vi "Get Bucket Notification Configuration.vi"(4 "Region":T1, 8 "error in (no error)":errorcluster, 9 "Bucket":string) -> (0 "error out":errorcluster, 3 "NotificationConfiguration":T2)   [LabVIEW 2015, in "LV Interface for Amazon S3.lvlib"]
doc: "This operation <B>returns the notification configuration</B> of a bucket. If notifications are not enabled on the bucket, the operation returns an empty NotificatonConfiguration element. <B>You must be the bucket owner to read the notification configuration</B> of a bucket. The bucket owner can use a bucket policy to grant permission to other users to read this configuration with the s3:GetBucketNotification permission."
uses:
  LV Interface for Amazon S3.lvlib
  Typedefs/AMZ_S3_NotificationConfiguration.ctl
  Typedefs/AMZ_S3_CompleteTopicConfiguration.ctl
  Typedefs/AMZ_S3_Event.ctl
  Typedefs/AMZ_S3_FilterRule.ctl
  Typedefs/AMZ_S3_CloudFunctionConfiguration.ctl
  Typedefs/AMZ_S3_QueueConfiguration.ctl
  Typedefs/AMZ_S3_LocationConstraint.ctl
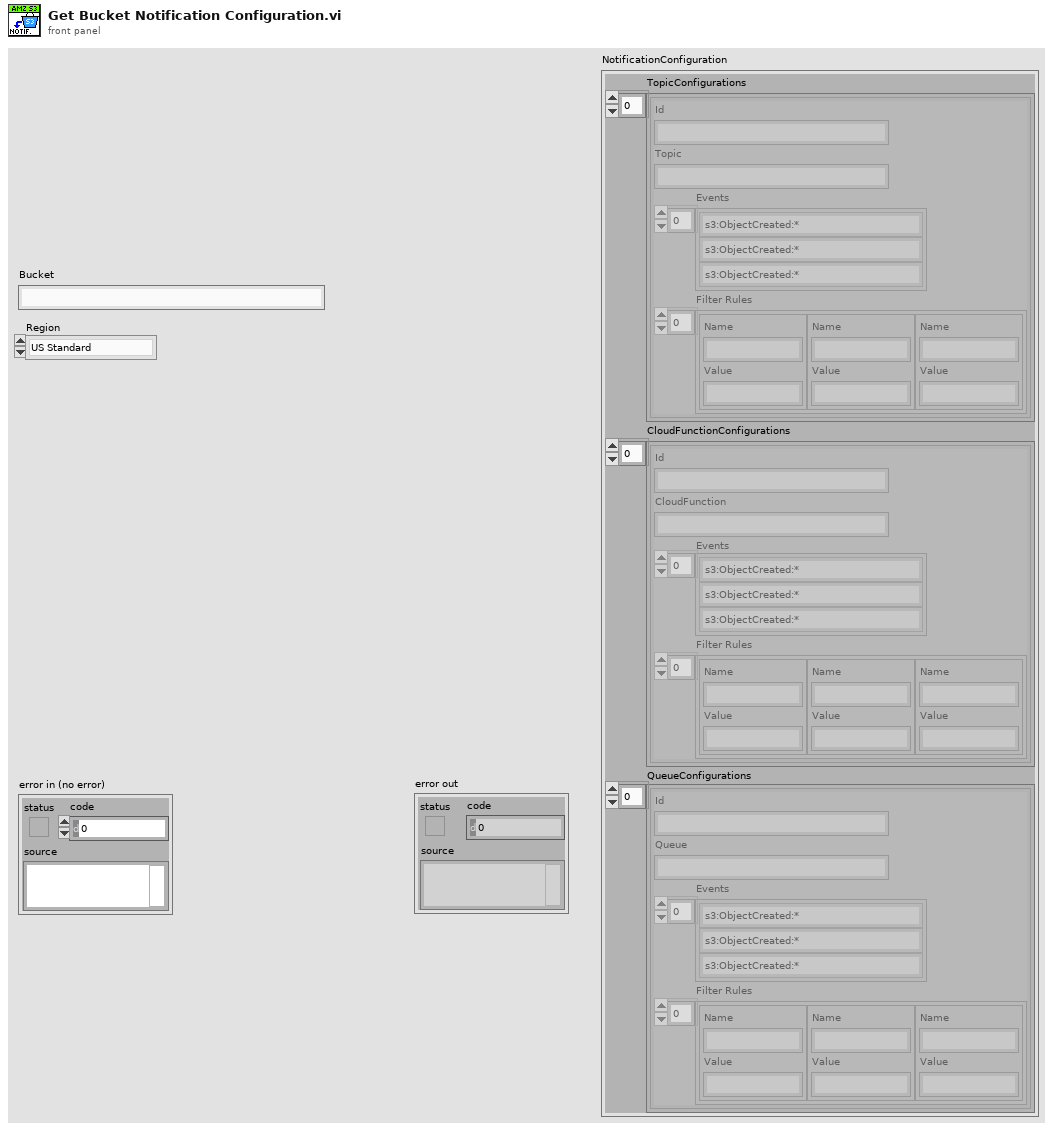
[diagram p1: front panel]
types:
  T1 = typedef "LV Interface for Amazon S3.lvlib/AMZ_S3_LocationConstraint.ctl" = enum16{"US Standard", "us-east-2", "us-west-1", "us-west-2", "ap-northeast-1", "ap-northeast-2", "ap-southeast-1", "ap-southeast-2", "ca-central-1", "eu-central-1", "eu-west-1", "eu-west-2", "sa-east-1"}
  T2 = typedef "LV Interface for Amazon S3.lvlib/AMZ_S3_NotificationConfiguration.ctl" = cluster{"TopicConfigurations":T3[], "CloudFunctionConfigurations":T6[], "QueueConfigurations":T7[]}
  T3 = typedef "LV Interface for Amazon S3.lvlib/AMZ_S3_CompleteTopicConfiguration.ctl" = cluster{"Id":string, "Topic":string, "Events":T4[], "Filter Rules":T5[]}
  T4 = typedef "LV Interface for Amazon S3.lvlib/AMZ_S3_Event.ctl" = enum16{"s3:ObjectCreated:*", "s3:ObjectCreated:Put", "s3:ObjectCreated:Post", "s3:ObjectCreated:Copy", "s3:ObjectCreated:CompleteMultipartUpload", "s3:ObjectRemoved:*", "s3:ObjectRemoved:Delete", "s3:ObjectRemoved:DeleteMarkerCreated", "s3:ReducedRedundancyLostObject"}
  T5 = typedef "LV Interface for Amazon S3.lvlib/AMZ_S3_FilterRule.ctl" = cluster{"Name":string, "Value":string}
  T6 = typedef "LV Interface for Amazon S3.lvlib/AMZ_S3_CloudFunctionConfiguration.ctl" = cluster{"Id":string, "CloudFunction":string, "Events":T4[], "Filter Rules":T5[]}
  T7 = typedef "LV Interface for Amazon S3.lvlib/AMZ_S3_QueueConfiguration.ctl" = cluster{"Id":string, "Queue":string, "Events":T4[], "Filter Rules":T5[]}
  T8 = typedef "LV Interface for Amazon S3.lvlib/AMZ_S3_Call Results.ctl" = enum16{"Success", "UndefinedError", "AccessDenied", "AccountProblem", "AmbiguousGrantByEmailAddress", "BadDigest", "BucketAlreadyExists", "BucketAlreadyOwnedByYou", "BucketNotEmpty", "CredentialsNotSupported", "CrossLocationLoggingProhibited", "EntityTooSmall", "EntityTooLarge", "ExpiredToken", "IllegalVersioningConfigurationException", "IncompleteBody", "IncorrectNumberOfFilesInPostRequest", "InlineDataTooLarge", "InternalError", "InvalidAccessKeyId", "InvalidAddressingHeader", "InvalidArgument", "InvalidBucketName", "InvalidDigest", "InvalidLocationConstraint", "InvalidPart", "InvalidPartOrder", "InvalidPayer", "InvalidPolicyDocument", "InvalidRange", "InvalidSecurity", "InvalidSOAPRequest", "InvalidStorageClass", "InvalidTargetBucketForLogging", "InvalidToken", "InvalidURI", "KeyTooLong", "MalformedACLError", "MalformedPOSTRequest", "MalformedXML", "MaxMessageLengthExceeded", "MaxPostPreDataLengthExceededError", "MetadataTooLarge", "MethodNotAllowed", "MissingAttachment", "MissingContentLength", "MissingRequestBodyError", "MissingSecurityElement", "MissingSecurityHeader", "NoLoggingStatusForKey", "NoSuchBucket", "NoSuchKey", "NoSuchUpload", "NoSuchVersion", "NotImplemented", "NotSignedUp", "OperationAborted", "PermanentRedirect", "PreconditionFailed", "Redirect", "RequestIsNotMultiPartContent", "RequestTimeout", "RequestTimeTooSkewed", "RequestTorrentOfBucketError", "SignatureDoesNotMatch", "SlowDown", "TemporaryRedirect", "TokenRefreshRequired", "TooManyBuckets", "UnexpectedContent", "UnresolvableGrantByEmailAddress", "UserKeyMustBeSpecified", "LabVIEWError"}
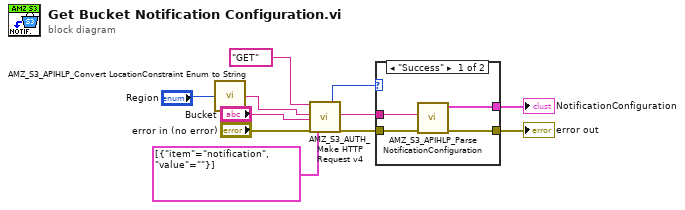
[diagram p0: block diagram]
diagram:
  n1 = call "AMZ_S3_APIHLP_Convert LocationConstraint Enum to String.vi"("Location"="Region") -> ("Location String"=w1:string)  [unwired: 4 in]
  n2 = call "AMZ_S3_AUTH_Make HTTP Request v4.vi"("HTTP-Verb"="GET", "Region"=w1, "Bucket"="Bucket", "error in"="error in (no error)", "request parameters"=cluster{"item":string, "value":string}[] [{"item"="notification", "value"=""}]) -> ("Call Result"=w5:T8, "response body"=w4:string, "error out"=w8:errorcluster)  [unwired: 11 in, 1 out]
  n3 = case shown="\"Success\"" w5 {
    tunnel: w8 -> [w15 w16]
    tunnel: w4 -> [w14 _]
    tunnel: [w13 _] -> w10
    tunnel: [w12 w16] -> w11
    frame "Success" {
      n4 = call "AMZ_S3_APIHLP_Parse NotificationConfiguration.vi"("error in (no error)"=w15, "Response body"=w14) -> ("error out"=w12:errorcluster, "NotificationConfiguration"=w13:T2)  [unwired: 8 in]
    }
    frame Default {
    }
  }
  "error out" <- w11
  "NotificationConfiguration" <- w10
